vi "countrate.vi"() -> ()   [LabVIEW 2015]
uses:
  <vilib>/Platform/TimedLoop/XDataNode/timing_clust.ctl
  <vilib>/Platform/TimedLoop/XDataNode/nitl_modes.ctl
  <vilib>/Platform/TimedLoop/XDataNode/wakeup.ctl
  <vilib>/Utility/file.llb/Write Delimited Spreadsheet (I64).vi
  <vilib>/platform/TimedLoop/XDataNode/XDataNode.xnode
  <vilib>/Platform/TimedLoop/XDataNode/XDNodeRunTimeDep.lvlib
panel:
  in  "total time":dbl=300.0
  in  "Period (s)":dbl=1.0
  out "Waveform Graph":i32[](graph)=[0, 47, 44, 50, 68, 51, 62, 72, 48, 45, 45, 74, 55, 72, 61, 65, 59, 55, 73, 56, 57, 63, 54, 59, 53, 55, 54, 50, 53, 50, 43, 50, 47, 45, 43, 52, 68, 50, 40, 55, 62, 42, 53, 55, 60, 50, 51, 42, 48, 35, 51, 33, 35, 43, 43, 54, 44, 35, 31, 42, 39, 46, 39, 42, 41, 52, 34, 42, 45, 40, 50, 38, 42, 30, 48, 34, 27, 36, 39, 32, 33, 36, 26, 31, 35, 25, 23, 25, 38, 26, 32, 34, 31, 25, 36, 27, 28, 26, 28, 34, 30, 28, 23, 30, 19, 29, 17, 16, 19, 24, 22, 19, 27, 18, 20, 23, 28, 29, 28, 29, 31, 21, 25, 28, 26, 19, 22, 27, 21, 14, 9, 20, 21, 15, 15, 18, 15, 18, 14, 14, 13, 13, 12, 26, 21, 26, 21, 12, 7, 20, 11, 18, 12, 12, 16, 12, 19, 13, 9, 15, 14, 10, 14, 13, 13, 16, 12, 22, 16, 17, 18, 11, 16, 5, 7, 9, 15, 9, 13, 14, 8, 10, 12, 10, 17, 14, 13, 12, 10, 11, 9, 9, 8, 19, 7, 19, 10, 8, 8, 15, 11, 15, 14, 9, 11, 10, 8, 8, 7, 9, 4, 12, 8, 4, 6, 10, 7, 18, 4, 6, 9, 5, 16, 4, 8, 7, 6, 9, 3, 8, 4, 7, 4, 4, 13, 7, 10, 7, 10, 8, 5, 3, 6, 11, 4, 5, 5, 6, 11, 2, 5, 6, 4, 12, 7, 7, 6, 13, 5, 4, 2, 7, 3, 7, 5, 6, 9, 2, 5, 0, 6, 7, 6, 9, 7, 4, 4, 5, 2, 6, 3, 6, 7, 6, 6, 7, 4, 7, 5, 8, 5, 7, 7, 10, 2, 3, 8, 5, 2, 11, 3]
  out "counts per second":dbl(knob)=3.0 scale=0.0..100.0
  in  "stop":bool
  # "Demo count rate VI for Physics 434"
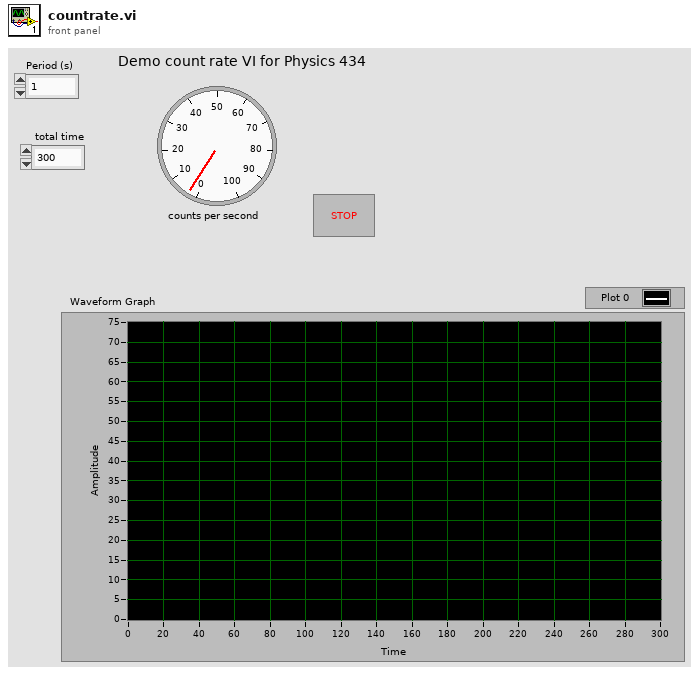
[diagram p1: front panel]
types:
  T1 = typedef "XDNodeRunTimeDep.lvlib/timing_clust.ctl" = cluster{"Expected End [f-1]":u64, "Actual End [f-1]":u64, "Finished Late? [f-1]":bool, "Expected End [i-1]":u64, "Actual End [i-1]":u64, "Finished Late? [i-1]":bool, "Expected Start [i]":u64, "Actual Start [i]":u64, "Expected Start [f]":u64, "Actual Start [f]":u64, "Source Name":string, "Structure Name":string, "Period":i64, "Deadline":i64, "Offset":i64, "Start":i64, "Priority":i32, "Timeout":i32, "Mode":T2, "Wakeup Reason":T3, "Error":errorcluster, "Source Type":string, "Secondary Source Type":string, "Global End Time":u64, "Global Start Time":u64, "Frame Duration":u64, "Iteration Duration":u64, "Assigned CPU":i32, "I/O Scan Engine Mode":u32}
  T2 = typedef "XDNodeRunTimeDep.lvlib/nitl_modes.ctl" = enum32{"No Change", "Process missed periods, maintain original phase", "Discard missed periods, maintain original phase", "Process missed periods, ignore original phase", "Discard missed periods, ignore original phase"}
  T3 = typedef "XDNodeRunTimeDep.lvlib/wakeup.ctl" = enum32{"Normal", "Aborted", "Asynchronous wakeup", "Timing source error", "Timed loop error", "Timeout"}
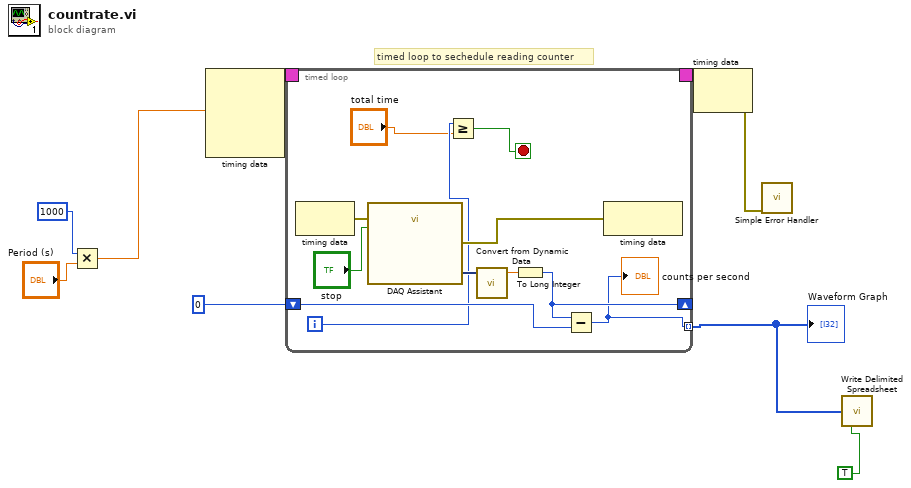
[diagram p0: block diagram]
diagram:
  # "timed loop to sechedule reading counter"
  n1 = Multiply(x=i64 1000 ("Period"), y="Period (s)") -> (x*y=w2:dbl)
  n2 = node-c288(w2) -> (w9:T1)  [unwired: 3 in]
  n3 = timed-loop {
    timing: w9 -> [_]
    timing-out: [_] -> w8
    shift-right: [w17] -> _
    shift-left: 0 -> [w19]
    tunnel: [w13] -> w5 mode=indexing
    i -> [w11]
    stop <- w12 stop-if-true
    n4 = node-c288() -> (w14:errorcluster)  [unwired: 1 in]
    n5 = call "DAQ Assistant"("error in"=w14, "stop (F)"="stop") -> ("data"=w20:dynamicdata, "error out"=w15:errorcluster)  [unwired: 14 in, 2 out]
    n6 = Greater Or Equal?(x=w11, y="total time") -> (x >= y?=w12:bool)
    n7 = call "Convert from Dynamic Data"("Dynamic Data Type"=w20) -> ("Scalar"=w16:dbl)  [unwired: 3 in]
    n8 = To Long Integer(number=w16) -> (32bit integer=w17:i32)
    n9 = Subtract(x=w17, y=w19) -> (x-y=w13:i32)
    "counts per second" <- w13
    n10 = node-c288(w15) -> ()  [unwired: 1 out]
  }
  "Waveform Graph" <- w5
  n11 = node-c288(w8) -> (w6:errorcluster)
  n12 = call <vilib>:"Simple Error Handler.vi"("error in (no error)"=w6) -> ()  [unwired: 4 in, 5 out]
  n13 = call-poly <vilib>:"Write Delimited Spreadsheet.vi"("1D data"=w5, "transpose? (F)"=TRUE) -> ()  [unwired: 12 in, 2 out]
